vi "Actor Core.vi"(8 "error in":errorcluster, 11 "Hotel Management Tool UI in":refnum<class "Hotel Management Tool UI.lvclass">) -> (0 "error out":errorcluster, 3 "Actor out":refnum<class "Actor.lvclass">)   [LabVIEW 2023, in "Hotel Management Tool UI.lvlib" / "Hotel Management Tool UI.lvclass"]
doc: "(<B>Filename</B>: Actor Framework.lvlib:Actor.lvclass:Actor Core.vi)\n\nReceives messages to the actor, reacts to them, and initiates any error handling that may shut the actor down.\n\nDescendant classes may override this VI to append parallel tasks for the actor to complete while it handles messages. Overrides use the Call Parent Class Method node."
uses:
  Hotel Management Tool UI.lvclass
  C:/Users/bhaghyaraj/Trainings/NI Actor Framework/SDLC/UI Base/UI Base/UI Base.lvclass
  C:/Program Files/National Instruments/LabVIEW 2023/vi.lib/ActorFramework/Actor/Actor.lvclass
  <vilib>/ActorFramework/Actor/Actor.lvclass
  <vilib>/ActorFramework/Actor/Actor.lvclass/Actor.ctl
  <vilib>/ActorFramework/Message Enqueuer/Message Enqueuer.lvclass/Message Enqueuer.ctl
  Hotel Management Tool UI.lvclass/Hotel Management Tool UI.ctl
  <vilib>/ActorFramework/Message Enqueuer/Init from Existing Queue.vi
  <vilib>/ActorFramework/Message Enqueuer/Enqueue.vi
  <vilib>/ActorFramework/Stop Msg/Stop Msg.lvclass
  C:/Program Files/National Instruments/LabVIEW 2023/vi.lib/ActorFramework/Message/Message.lvclass
  Hotel Management Tool UI Messages/Launch Rooms Manager Msg/Launch Rooms Manager Msg.lvclass
  <vilib>/ActorFramework/Message Priority Queue/Priority Enqueue.vi
  <vilib>/ActorFramework/Message Enqueuer/Message Enqueuer.lvclass
  UI Base/UI Base/UI Base.lvclass
panel:
  in  "Launch Rooms Manager":bool
  # "Welcome To Hotel Taj"
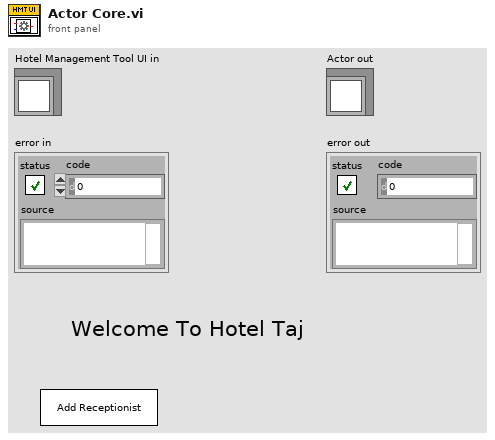
[diagram p1: front panel]
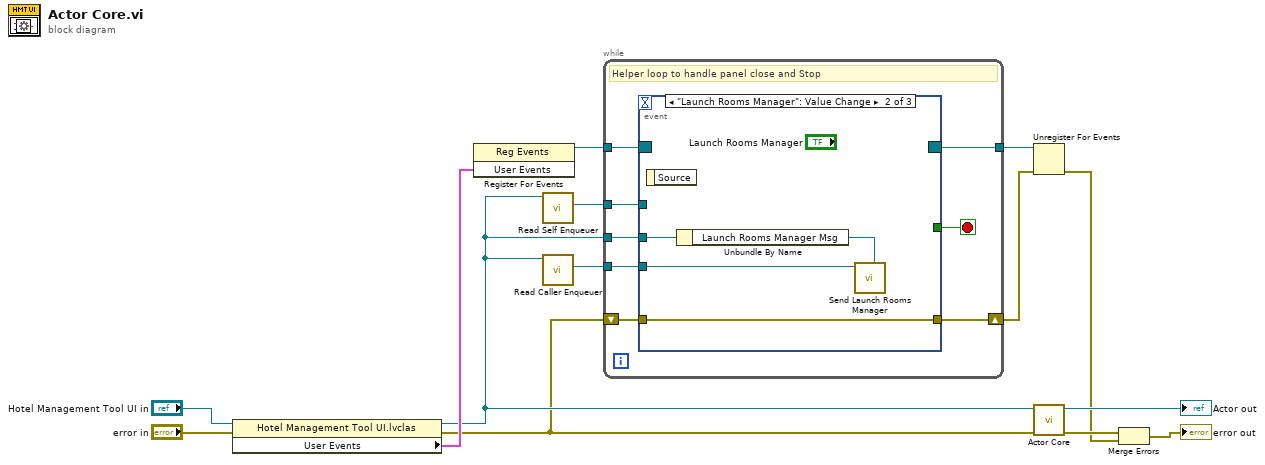
[diagram p0: block diagram]
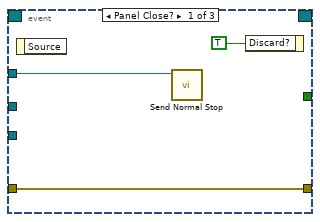
[diagram p2: hidden frame]
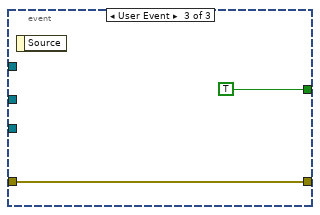
[diagram p3: hidden frame]
diagram:
  n1 = property class="Hotel Management Tool UI.lvclas"(reference="Hotel Management Tool UI in", error in="error in") -> (reference out=w3:refnum<class "Hotel Management Tool UI.lvclass">, error out=w2:errorcluster, "User Events"=w7:cluster{"Stop":refnum<user-event>})
  n2 = register-events(w7) -> (reference out=w10:refnum<event-registration>)  [unwired: 2 in, 1 out]
  n3 = call <vilib>:"Read Self Enqueuer.vi"("Actor"=w3) -> ("Self Enqueuer"=w9:refnum<class "Message Enqueuer.lvclass">)  [unwired: 10 in]
  n4 = call <vilib>:"Read Caller Enqueuer.vi"("Actor"=w3) -> ("Caller Enqueuer"=w4:refnum<class "Message Enqueuer.lvclass">)  [unwired: 10 in]
  n5 = while {
    tunnel: w9 -> [w22]
    tunnel: w10 -> [w21]
    tunnel: [w19] -> w11
    tunnel: w4 -> [w18]
    tunnel: w3 -> [w17]
    shift-right: [w15] -> w1
    shift-left: w2 -> [w16]
    stop <- w20 stop-if-true
    # "Helper loop to handle panel close and Stop"
    n6 = event shown="[1] \"Launch Rooms Manager\": Value Change" {
      selector: w21 -> [_ _ _]
      dyn-events: [_ _ _] -> w19
      timeout: _ -> [_ _ _]
      tunnel: w22 -> [w24 _ _]
      tunnel: [_ _ TRUE] -> w20
      tunnel: w18 -> [_ w29 _]
      tunnel: w17 -> [_ w28 _]
      tunnel: w16 -> [w23 w26 w30]
      tunnel: [w23 w26 w30] -> w15
      event Panel Close? {
        n7 = event-data() -> ()  [unwired: 1 in, 1 out]
        n8 = call <vilib>:"Send Normal Stop.vi"("Message Enqueuer"=w24) -> ()  [unwired: 10 in, 1 out]
        n9 = event-data("Discard?"=TRUE) -> ()  [unwired: 1 in, 1 out]
      }
      event "Launch Rooms Manager": Value Change {
        n10 = event-data() -> ()  [unwired: 1 in, 1 out]
        n11 = Unbundle By Name(w28) -> ("Launch Rooms Manager Msg"=w27:refnum<class "Launch Rooms Manager Msg.lvclass">)
        n12 = call "Send Launch Rooms Manager.vi"("Message Type"=w27, "Message Enqueuer"=w29) -> ()  [unwired: 8 in, 2 out]
      }
      event User Event {
        n13 = event-data() -> ()  [unwired: 1 in, 1 out]
      }
    }
  }
  n14 = Unregister For Events(event registration refnum=w11, error in=w1) -> (error out=w5:errorcluster)
  n15 = call-parent "Actor Core.vi"("error in"=w2, "Actor in"=w3) -> ("error out"=w14:errorcluster, "Actor out"=→"Actor out":refnum<class "Actor.lvclass">)  [unwired: 8 in]
  n16 = Merge Errors(w14, w5) -> (→"error out":errorcluster)
